vi "MovCor-QueueStartStop from anywhere.vi"(8 "error in (no error)":errorcluster, 11 "Start/Stop":T1=enum."STOP") -> (0 "error out":errorcluster)   [LabVIEW 2020]
uses:
  Typedefs/Top level VI states.ctl
  Global Variables/General Globals.vi
  Typedefs/Start-Stop Enum.ctl
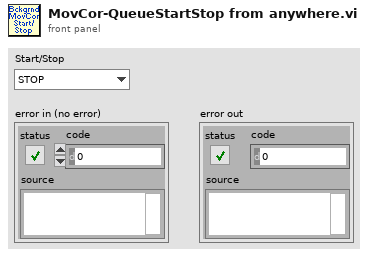
[diagram p1: front panel]
types:
  T1 = typedef "Start-Stop Enum.ctl" = enum16{"START", "STOP"}
  T2 = typedef "Top level VI states.ctl" = enum16{"None", "Initialise UI", "<STACK PROTOCOL STATES>", "AOL Zstack-START", "AOL Zstack-STOP", "Motor Zstack-START", "Motor Zstack-STOP", "<ACQUISITION PROTOCOL STATES> ", "Functional Acquisition-START", "Functional Acquisition-STOP", "Single Plane Acquisition-START", "Single Plane Acquisition-STOP", "Volume Acquisition-START", "Volume Acquisition-STOP", "<LIVE IMAGING PROTOCOL STATES>", "Live Imaging-START", "Live Imaging-STOP", "Live Plane Imaging-START", "Live Plane Imaging-STOP", "Live Volume Imaging-START", "Live Volume Imaging-STOP", "<MOVEMENT CORRECTION PROTOCOL STATES>", "EXIT"}
  T3 = typedef "Top level VI states.ctl" = enum16{"None", "Initialise UI", "<STACK PROTOCOL STATES>", "AOL Zstack-START", "AOL Zstack-STOP", "Motor Zstack-START", "Motor Zstack-STOP", "<ACQUISITION PROTOCOL STATES> ", "Functional Acquisition-START", "Functional Acquisition-STOP", "Single Plane Acquisition-START", "Single Plane Acquisition-STOP", "Volume Acquisition-START", "Volume Acquisition-STOP", "<LIVE IMAGING PROTOCOL STATES>", "Live Imaging-START", "Live Imaging-STOP", "Live Plane Imaging-START", "Live Plane Imaging-STOP", "Live Volume Imaging-START", "Live Volume Imaging-STOP", "<MOVEMENT CORRECTION PROTOCOL STATES>", "Background MovCor-START", "Background MovCor-STOP", "EXIT"}
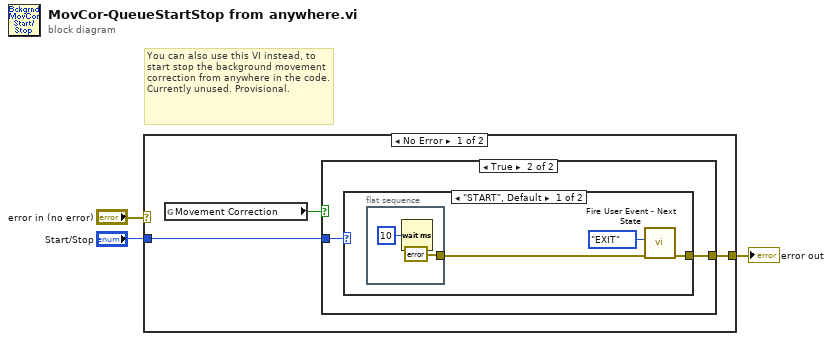
[diagram p0: block diagram]
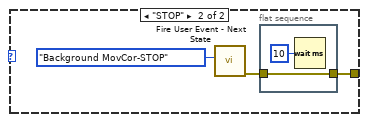
[diagram p3: hidden frame]
diagram:
  # "You can also use this VI instead, to start stop the background movement correction from anywhere in the code. Currently unused. Provisional."
  n1 = case shown="No Error" "error in (no error)" {
    selector: "error in (no error)" -> [_ w19]
    tunnel: [w6 w19] -> w1
    tunnel: "Start/Stop" -> [w5 _]
    frame No Error {
      n2 = global read "General Globals.vi" "Movement Correction"() -> (w4:bool)
      n3 = case shown="True" w4 {
        tunnel: [_ w8] -> w6
        tunnel: w5 -> [_ w7]
        frame False {
        }
        frame True {
          n4 = case shown="\"START\", Default" w7 {
            tunnel: [w10 w14] -> w8
            frame "START", Default {
              n5 = flat-sequence {
                tunnel: [errorcluster {"status"=FALSE, "code"=0, "source"=""} ("Error Out")] -> w9
                frame #0 {
                  n6 = Wait (ms)(milliseconds to wait=u32 10) -> ()  [unwired: 1 out]
                }
              }
              n7 = call "Fire User Event - Next State.vi"("Error In"=w9, "\"UI Handler loop\" case to execute"=Top_level_VI_states."EXIT" ("\"UI Handler loop\" case to execute")) -> ("Error Out"=w10:errorcluster)  [unwired: 9 in]
            }
            frame "STOP" {
              n8 = call "Fire User Event - Next State.vi"("\"UI Handler loop\" case to execute"=Top_level_VI_states."Background MovCor-STOP" ("\"UI Handler loop\" case to execute")) -> ("Error Out"=w15:errorcluster)  [unwired: 10 in]
              n9 = flat-sequence {
                tunnel: [w17] -> w14
                tunnel: w15 -> [w17]
                frame #0 {
                  n10 = Wait (ms)(milliseconds to wait=u32 10) -> ()  [unwired: 1 out]
                }
              }
            }
          }
        }
      }
    }
    frame Error {
    }
  }
  "error out" <- w1
